vi "Read Flow.vi"(8 "error in (no error)":errorcluster, 11 "MFC Actor.lvlib:MFC.lvclass":refnum<class "MFC.lvclass">) -> (0 "error out":errorcluster, 3 "Actor out":refnum<class "Actor.lvclass">)   [LabVIEW 2018, in "MFC Actor.lvlib" / "MFC.lvclass"]
uses:
  MFC.lvclass
  <vilib>/ActorFramework/Actor/Actor.lvclass
  C:/Program Files/National Instruments/LabVIEW 2018/vi.lib/ActorFramework/Actor/Actor.lvclass
  MFC.lvclass/MFC.ctl
  <instrlib>/Sierra Instruments Smart-Trak 100 Series/Sierra Instruments Smart-Trak 100 Series.lvlib
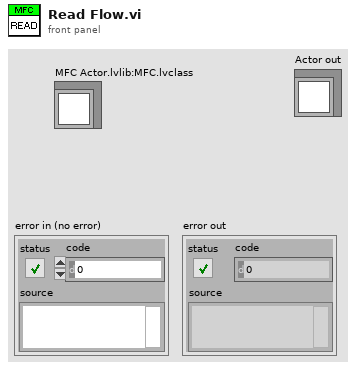
[diagram p1: front panel]
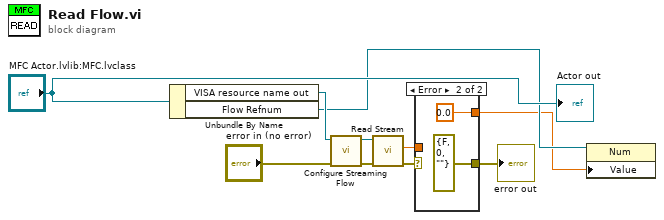
[diagram p0: block diagram]
diagram:
  n1 = Unbundle By Name("MFC Actor.lvlib:MFC.lvclass") -> ("VISA resource name out"=w5:refnum<visa-resource-name>, "Flow Refnum"=w2:refnum<vi>)
  n2 = call <instrlib>:"Configure Streaming Flow.vi"("error in (no error)"="error in (no error)", "VISA resource name"=w5) -> ("error out"=w7:errorcluster, "VISA resource name out"=w8:refnum<visa-resource-name>)  [unwired: 8 in]
  n3 = call <instrlib>:"Read Stream.vi"("error in (no error)"=w7, "VISA resource name"=w8) -> ("error out"=w3:errorcluster, "Flow"=w4:dbl)  [unwired: 6 in, 2 out]
  n4 = case shown="Error" w3 {
    selector: w3 -> [w12 _]
    tunnel: [w12 errorcluster {"status"=FALSE, "code"=0, "source"=""} ("error IO")] -> w10
    tunnel: w4 -> [w11 _]
    tunnel: [w11 0.0 ("data")] -> w1
    frame No Error {
    }
    frame Error {
    }
  }
  "error out" <- w10
  n5 = property class="Num"(reference=w2, "Value"=w1) -> ()  [unwired: 1 in, 2 out]
  "Actor out" <- "MFC Actor.lvlib:MFC.lvclass"
